vi "Waveform point address control.vi"(4 "Input Valid":bool, 6 "Total elements":u32, 8 "Elements wrote in":u32) -> (1 "All points written":bool, 3 "Elements wrote out":u32)   [LabVIEW 2015]
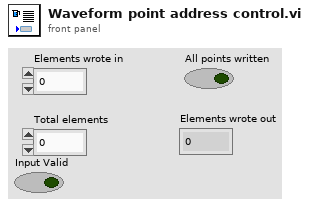
[diagram p1: front panel]
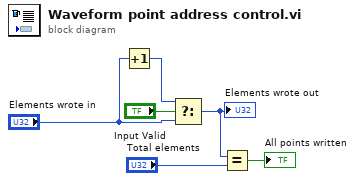
[diagram p0: block diagram]
diagram:
  n1 = Increment(x="Elements wrote in") -> (x+1=w2:u32)
  n2 = Select(t=w2, s="Input Valid", f="Elements wrote in") -> (s? t:f=w5:u32)
  "Elements wrote out" <- w5
  n3 = Equal?(x=w5, y="Total elements") -> (x = y?=→"All points written":bool)
